vi "Event Messenger Channel Lesson 4a (right way).vi"() -> ()   [LabVIEW 2019]
doc: "Lesson 4a shows the right way to have one Event Messenger channel wire trigger two separate Event structures."
uses:
  <extravilib>/ChannelInstances/Event Messenger-i32/Instantiate.vi
  <extravilib>/ChannelInstances/Event Messenger-i32/))Channel.vi
  <extravilib>/ChannelInstances/Event Messenger-i32.lvlib
panel:
  out "Consumer Beta":i32
  out "Producer":i32
  out "Consumer Alpha":i32
  in  "Stop":bool
  # "Overview: This VI demonstrates how to use the Event Messenger channel wire.\n\nLesson 4a shows the right way to have one Event Messenger channel wire trigger two separate Event structures.\n\nInstructions:\n1. Run the VI. Notice that the Producer and both consumers run at about the same rate.\n2. Notice that each time the Producer loop writes data to the channel, it is received by both Consumer loops.\n3. Press the Stop button to stop the VI.\n4. Open the block diagram. Review the comments there to see how this VI works."
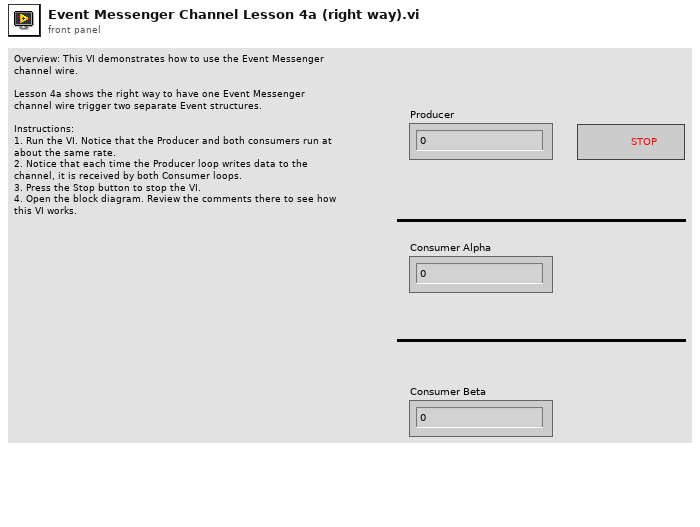
[diagram p1: front panel]
types:
  T1 = typedef "Event Messenger-i32.lvlib/))Channel.ctl" = refnum<queue>
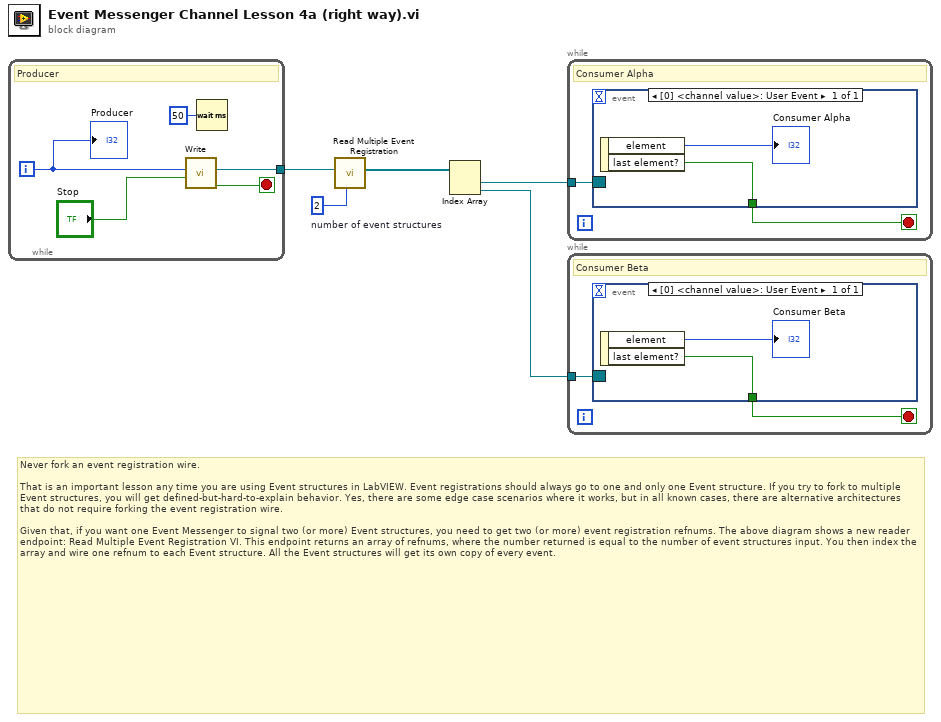
[diagram p0: block diagram]
diagram:
  w4 = u16 2  # number of event structures
  # "Never fork an event registration wire. \n\nThat is an important lesson any time you are using Event structures in LabVIEW. Event registrations should always go to one and only one Event structure. If you try to fork to multiple Event structures, you will get defined-but-hard-to-explain behavior. Yes, there are some edge case scenarios where it works, but in all known cases, there are alternative architectures that do not require forking the event registration wire. \n\nGiven that, if you want one Event Messenger to signal two (or more) Event structures, you need to get two (or more) event registration refnums. The above diagram shows a new reader endpoint: Read Multiple Event Registration VI. This endpoint returns an array of refnums, where the number returned is equal to the number of event structures input. You then index the array and wire one refnum to each Event structure. All the Event structures will get its own copy of every event."
  n1 = while {
    tunnel: [w7] -> w5
    i -> [w10]
    stop <- w9 stop-if-true
    # "Producer"
    n2 = call <extravilib>:"Write.vi"("last element? (F)"="Stop", "element"=w10) -> ("done?"=w9:bool, "channel"=w7:T1)  [unwired: 8 in]
    n3 = Wait (ms)(milliseconds to wait=u32 50) -> ()  [unwired: 1 out]
    "Producer" <- w10
  }
  n4 = call <extravilib>:"Read Multiple Event Registration.vi"("number of event structures"=w4, "channel"=w5) -> ("event registration refnums"=w3:refnum<event-registration>[])  [unwired: 9 in]
  n5 = Index Array(array=w3) -> (element #1=w2:refnum<event-registration>, element #2=w1:refnum<event-registration>)  [unwired: 2 in]
  n6 = while {
    tunnel: w2 -> [w12]
    stop <- w11 stop-if-true
    # "Consumer Alpha"
    n7 = event shown="[0] <channel value>: User Event" {
      selector: w12 -> [_]
      dyn-events: _ -> [_]
      timeout: _ -> [_]
      tunnel: [w13] -> w11
      event User Event {
        n8 = event-data() -> ("element"=→"Consumer Alpha":i32, "last element?"=w13:bool)  [unwired: 1 in]
      }
    }
  }
  n9 = while {
    tunnel: w1 -> [w16]
    stop <- w15 stop-if-true
    # "Consumer Beta"
    n10 = event shown="[0] <channel value>: User Event" {
      selector: w16 -> [_]
      dyn-events: _ -> [_]
      timeout: _ -> [_]
      tunnel: [w18] -> w15
      event User Event {
        n11 = event-data() -> ("element"=→"Consumer Beta":i32, "last element?"=w18:bool)  [unwired: 1 in]
      }
    }
  }
